vi "logHardpointActuatorInfo.vi"(8 "error in (no error)":errorcluster, 10 "EventHardpointActuatorInfo":T1, 11 "M1M3SAL in":refnum<class "M1M3SAL.lvclass">) -> (0 "error out":errorcluster, 3 "M1M3SAL out":refnum<class "M1M3SAL.lvclass">)   [LabVIEW 2016, in "M1M3SupportCommunicator.lvlib" / "M1M3SAL.lvclass"]
uses:
  M1M3SAL.lvclass
  DataTypes/Topics/EventHardpointActuatorInfo.ctl
  DataTypes/Topics/Parts/Timestamp.ctl
  DataTypes/MessageHeader.ctl
  DataTypes/MessageTypes.ctl
  DataTypes/MessageTopics.ctl
  M1M3SAL.lvclass/M1M3SAL.ctl
  writeU8.vi
  writeSGL.vi
  writeI64.vi
  writeBoolean.vi
  M1M3SupportCommunicator.lvlib
  DataTypes/Topics/M1M3SupportTopics.lvlib
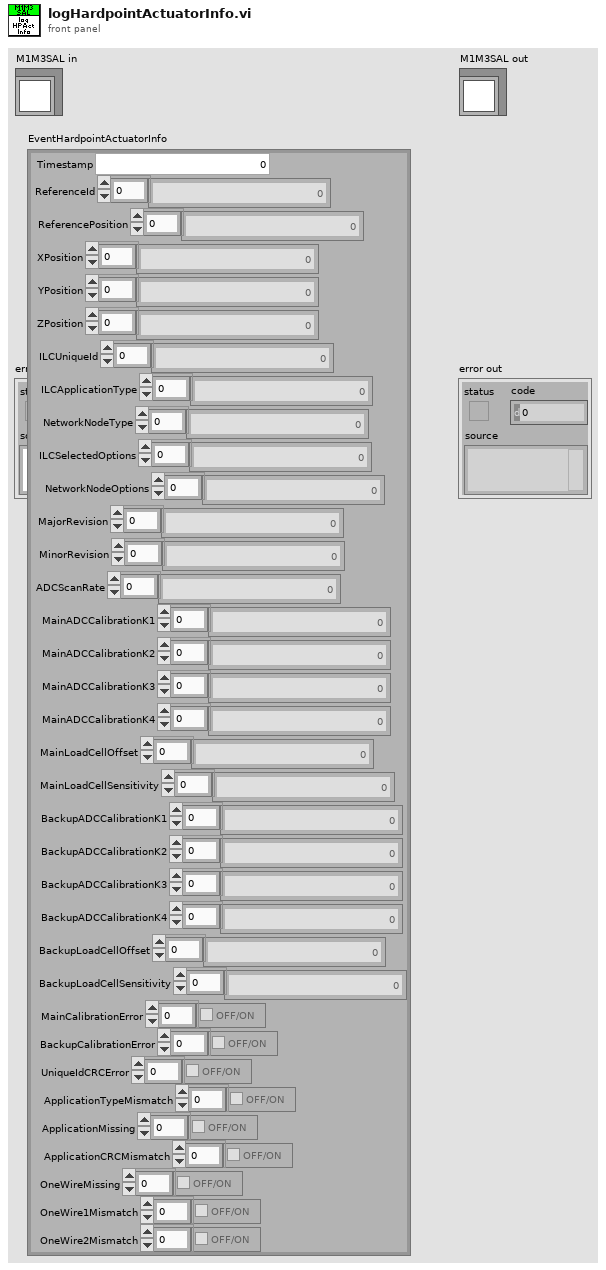
[diagram p1: front panel]
types:
  T1 = typedef "M1M3SupportTopics.lvlib/EventHardpointActuatorInfo.ctl" = cluster{"Timestamp":T2, "ReferenceId":i32[], "ReferencePosition":i32[], "XPosition":sgl[], "YPosition":sgl[], "ZPosition":sgl[], "ILCUniqueId":i64[], "ILCApplicationType":u8[], "NetworkNodeType":u8[], "ILCSelectedOptions":u8[], "NetworkNodeOptions":u8[], "MajorRevision":u8[], "MinorRevision":u8[], "ADCScanRate":u8[], "MainADCCalibrationK1":sgl[], "MainADCCalibrationK2":sgl[], "MainADCCalibrationK3":sgl[], "MainADCCalibrationK4":sgl[], "MainLoadCellOffset":sgl[], "MainLoadCellSensitivity":sgl[], "BackupADCCalibrationK1":sgl[], "BackupADCCalibrationK2":sgl[], "BackupADCCalibrationK3":sgl[], "BackupADCCalibrationK4":sgl[], "BackupLoadCellOffset":sgl[], "BackupLoadCellSensitivity":sgl[], "MainCalibrationError":bool[], "BackupCalibrationError":bool[], "UniqueIdCRCError":bool[], "ApplicationTypeMismatch":bool[], "ApplicationMissing":bool[], "ApplicationCRCMismatch":bool[], "OneWireMissing":bool[], "OneWire1Mismatch":bool[], "OneWire2Mismatch":bool[]}
  T2 = typedef "M1M3SupportTopics.lvlib/Timestamp.ctl" = dbl
  T3 = typedef "M1M3SupportCommunicator.lvlib/MessageHeader.ctl" = cluster{"Type":T4, "Topic":T5, "Size":i32}
  T4 = typedef "M1M3SupportCommunicator.lvlib/MessageTypes.ctl" = enum8{"None", "PutSample", "GetNextSample", "LogEvent", "GetEvent", "IssueCommand", "CommandId", "WaitForCompletion", "AcceptCommand", "AckCommand"}
  T5 = typedef "M1M3SupportCommunicator.lvlib/MessageTopics.ctl" = enum8{"None", "ForceActuatorData", "MirrorForceData", "HardpointData", "AirData", "DynamicData", "FPGAData", "IMSData", "ForceActuatorStatus", "ElevationData", "HardpointStatus", "HardpointActuatorChase", "AirStatus", "ForceActuatorSafetyChecks", "ForceActuatorTest", "ActuatorBroadcastCounter", "StatusChecks", "CellChecks", "HardpointActuatorBreakaway", "RaiseMirrorComplete", "ILCCommunication", "ElevationAngleChecks", "DetailedState", "ServoLoops", "ForceActuatorInfo", "LowerMirrorComplete", "HardpointActuatorInfo", "SettingsApplied", "ErrorCode", "StartupChecks", "SummaryState", "SettingVersions", "ActuatorTestStatus", "AppliedSettingsMatchStart", "Enable", "EnterMaintenance", "Standby", "AbortLowerM1M3", "ApplyAberrationByForces", "ApplyAOSCorrectionByBendingModes", "ClearAOSCorrection", "Start", "RaiseM1M3", "TestForceActuator", "LowerM1M3", "ApplyAOSCorrectionByForces", "Disable", "ApplyAberationByBendingMode", "TestHardpoint", "ManipulateM1M3", "ClearAberration", "Exit", "TestAir", "AbortRaiseM1M3", "MoveHardpointActuators", "ExitMaintenance", "Shutdown"}
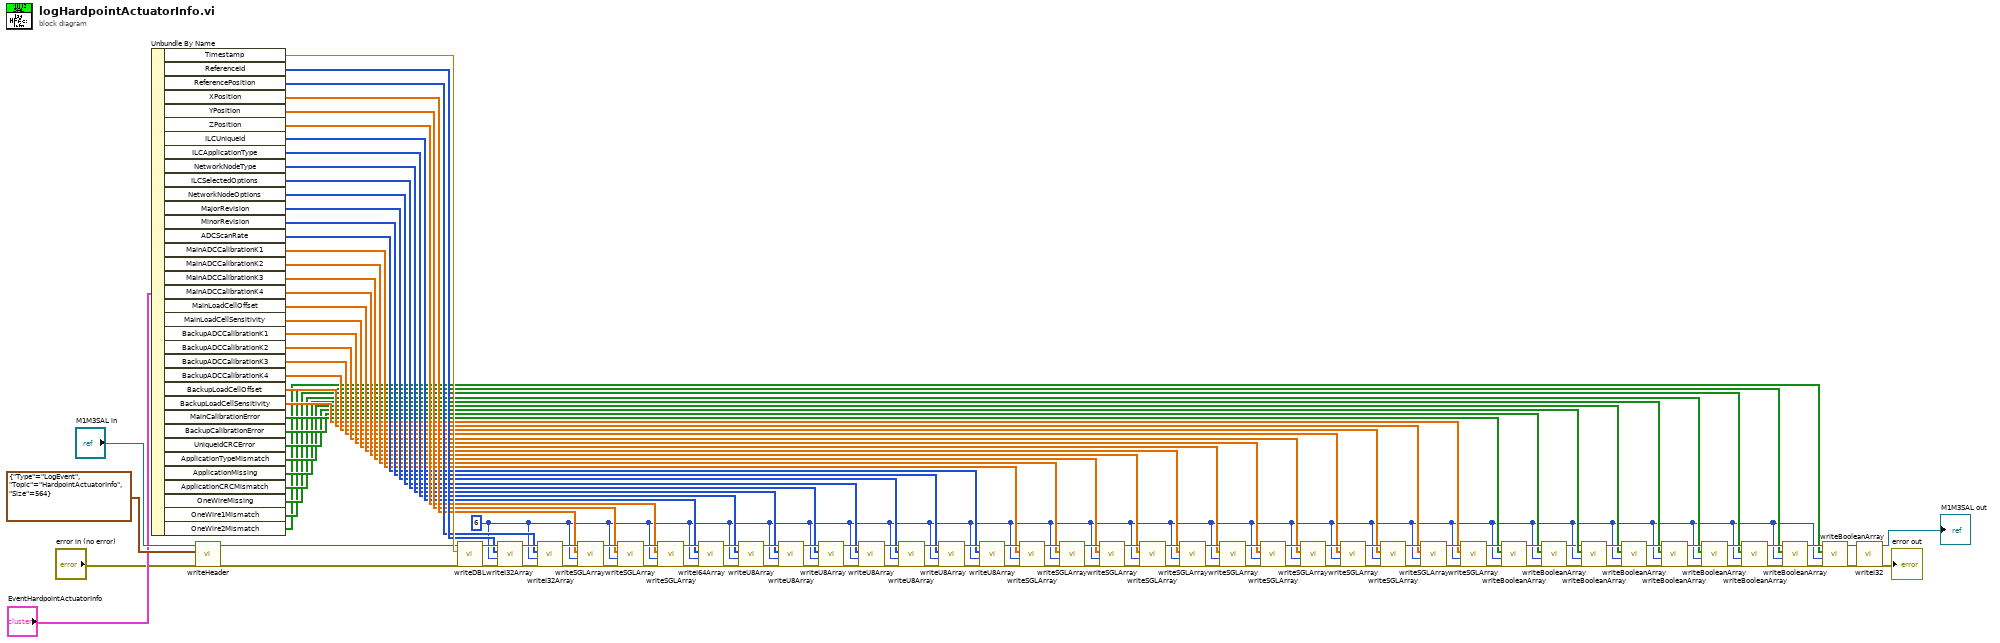
[diagram p0: block diagram]
diagram:
  w4 = 6
  n1 = Unbundle By Name("EventHardpointActuatorInfo") -> ("Timestamp"=w41:T2, "ReferenceId"=w40:i32[], "ReferencePosition"=w39:i32[], "XPosition"=w38:sgl[], "YPosition"=w37:sgl[], "ZPosition"=w36:sgl[], "ILCUniqueId"=w35:i64[], "ILCApplicationType"=w34:u8[], "NetworkNodeType"=w33:u8[], "ILCSelectedOptions"=w32:u8[], "NetworkNodeOptions"=w31:u8[], "MajorRevision"=w30:u8[], "MinorRevision"=w29:u8[], "ADCScanRate"=w28:u8[], "MainADCCalibrationK1"=w27:sgl[], "MainADCCalibrationK2"=w26:sgl[], "MainADCCalibrationK3"=w25:sgl[], "MainADCCalibrationK4"=w24:sgl[], "MainLoadCellOffset"=w23:sgl[], "MainLoadCellSensitivity"=w22:sgl[], "BackupADCCalibrationK1"=w21:sgl[], "BackupADCCalibrationK2"=w20:sgl[], "BackupADCCalibrationK3"=w19:sgl[], "BackupADCCalibrationK4"=w18:sgl[], "BackupLoadCellOffset"=w17:sgl[], "BackupLoadCellSensitivity"=w16:sgl[], "MainCalibrationError"=w15:bool[], "BackupCalibrationError"=w14:bool[], "UniqueIdCRCError"=w13:bool[], "ApplicationTypeMismatch"=w10:bool[], "ApplicationMissing"=w9:bool[], "ApplicationCRCMismatch"=w8:bool[], "OneWireMissing"=w7:bool[], "OneWire1Mismatch"=w6:bool[], "OneWire2Mismatch"=w5:bool[])
  n2 = call "writeHeader.vi"("error in (no error)"="error in (no error)", "MessageHeader"=T3 {"Type"=enum."LogEvent", "Topic"=enum."HardpointActuatorInfo", "Size"=564}, "M1M3SAL in"="M1M3SAL in") -> ("error out"=w2:errorcluster, "M1M3SAL out"=w3:refnum<class "M1M3SAL.lvclass">)  [unwired: 7 in]
  n3 = call "writeDBL.vi"("error in (no error)"=w2, "Input"=w41, "M1M3SAL in"=w3) -> ("error out"=w107:errorcluster, "M1M3SAL out"=w106:refnum<class "M1M3SAL.lvclass">)  [unwired: 7 in]
  n4 = call "writeI32Array.vi"("error in (no error)"=w107, "Length"=w4, "Input"=w40, "M1M3SAL in"=w106) -> ("error out"=w111:errorcluster, "M1M3SAL out"=w110:refnum<class "M1M3SAL.lvclass">)  [unwired: 6 in]
  n5 = call "writeI32Array.vi"("error in (no error)"=w111, "Length"=w4, "Input"=w39, "M1M3SAL in"=w110) -> ("error out"=w108:errorcluster, "M1M3SAL out"=w109:refnum<class "M1M3SAL.lvclass">)  [unwired: 6 in]
  n6 = call "writeSGLArray.vi"("error in (no error)"=w108, "Length"=w4, "Input"=w38, "M1M3SAL in"=w109) -> ("error out"=w105:errorcluster, "M1M3SAL out"=w104:refnum<class "M1M3SAL.lvclass">)  [unwired: 6 in]
  n7 = call "writeSGLArray.vi"("error in (no error)"=w105, "Length"=w4, "Input"=w37, "M1M3SAL in"=w104) -> ("error out"=w103:errorcluster, "M1M3SAL out"=w102:refnum<class "M1M3SAL.lvclass">)  [unwired: 6 in]
  n8 = call "writeSGLArray.vi"("error in (no error)"=w103, "Length"=w4, "Input"=w36, "M1M3SAL in"=w102) -> ("error out"=w100:errorcluster, "M1M3SAL out"=w101:refnum<class "M1M3SAL.lvclass">)  [unwired: 6 in]
  n9 = call "writeI64Array.vi"("error in (no error)"=w100, "Length"=w4, "Input"=w35, "M1M3SAL in"=w101) -> ("error out"=w98:errorcluster, "M1M3SAL out"=w99:refnum<class "M1M3SAL.lvclass">)  [unwired: 6 in]
  n10 = call "writeU8Array.vi"("error in (no error)"=w98, "Length"=w4, "Input"=w34, "M1M3SAL in"=w99) -> ("error out"=w97:errorcluster, "M1M3SAL out"=w96:refnum<class "M1M3SAL.lvclass">)  [unwired: 6 in]
  n11 = call "writeU8Array.vi"("error in (no error)"=w97, "Length"=w4, "Input"=w33, "M1M3SAL in"=w96) -> ("error out"=w95:errorcluster, "M1M3SAL out"=w94:refnum<class "M1M3SAL.lvclass">)  [unwired: 6 in]
  n12 = call "writeU8Array.vi"("error in (no error)"=w95, "Length"=w4, "Input"=w32, "M1M3SAL in"=w94) -> ("error out"=w93:errorcluster, "M1M3SAL out"=w92:refnum<class "M1M3SAL.lvclass">)  [unwired: 6 in]
  n13 = call "writeU8Array.vi"("error in (no error)"=w93, "Length"=w4, "Input"=w31, "M1M3SAL in"=w92) -> ("error out"=w91:errorcluster, "M1M3SAL out"=w90:refnum<class "M1M3SAL.lvclass">)  [unwired: 6 in]
  n14 = call "writeU8Array.vi"("error in (no error)"=w91, "Length"=w4, "Input"=w30, "M1M3SAL in"=w90) -> ("error out"=w89:errorcluster, "M1M3SAL out"=w88:refnum<class "M1M3SAL.lvclass">)  [unwired: 6 in]
  n15 = call "writeU8Array.vi"("error in (no error)"=w89, "Length"=w4, "Input"=w29, "M1M3SAL in"=w88) -> ("error out"=w87:errorcluster, "M1M3SAL out"=w86:refnum<class "M1M3SAL.lvclass">)  [unwired: 6 in]
  n16 = call "writeU8Array.vi"("error in (no error)"=w87, "Length"=w4, "Input"=w28, "M1M3SAL in"=w86) -> ("error out"=w85:errorcluster, "M1M3SAL out"=w84:refnum<class "M1M3SAL.lvclass">)  [unwired: 6 in]
  n17 = call "writeSGLArray.vi"("error in (no error)"=w85, "Length"=w4, "Input"=w27, "M1M3SAL in"=w84) -> ("error out"=w83:errorcluster, "M1M3SAL out"=w82:refnum<class "M1M3SAL.lvclass">)  [unwired: 6 in]
  n18 = call "writeSGLArray.vi"("error in (no error)"=w83, "Length"=w4, "Input"=w26, "M1M3SAL in"=w82) -> ("error out"=w81:errorcluster, "M1M3SAL out"=w80:refnum<class "M1M3SAL.lvclass">)  [unwired: 6 in]
  n19 = call "writeSGLArray.vi"("error in (no error)"=w81, "Length"=w4, "Input"=w25, "M1M3SAL in"=w80) -> ("error out"=w79:errorcluster, "M1M3SAL out"=w78:refnum<class "M1M3SAL.lvclass">)  [unwired: 6 in]
  n20 = call "writeSGLArray.vi"("error in (no error)"=w79, "Length"=w4, "Input"=w24, "M1M3SAL in"=w78) -> ("error out"=w77:errorcluster, "M1M3SAL out"=w76:refnum<class "M1M3SAL.lvclass">)  [unwired: 6 in]
  n21 = call "writeSGLArray.vi"("error in (no error)"=w77, "Length"=w4, "Input"=w23, "M1M3SAL in"=w76) -> ("error out"=w75:errorcluster, "M1M3SAL out"=w74:refnum<class "M1M3SAL.lvclass">)  [unwired: 6 in]
  n22 = call "writeSGLArray.vi"("error in (no error)"=w75, "Length"=w4, "Input"=w22, "M1M3SAL in"=w74) -> ("error out"=w73:errorcluster, "M1M3SAL out"=w72:refnum<class "M1M3SAL.lvclass">)  [unwired: 6 in]
  n23 = call "writeSGLArray.vi"("error in (no error)"=w73, "Length"=w4, "Input"=w21, "M1M3SAL in"=w72) -> ("error out"=w71:errorcluster, "M1M3SAL out"=w70:refnum<class "M1M3SAL.lvclass">)  [unwired: 6 in]
  n24 = call "writeSGLArray.vi"("error in (no error)"=w71, "Length"=w4, "Input"=w20, "M1M3SAL in"=w70) -> ("error out"=w69:errorcluster, "M1M3SAL out"=w68:refnum<class "M1M3SAL.lvclass">)  [unwired: 6 in]
  n25 = call "writeSGLArray.vi"("error in (no error)"=w69, "Length"=w4, "Input"=w19, "M1M3SAL in"=w68) -> ("error out"=w67:errorcluster, "M1M3SAL out"=w66:refnum<class "M1M3SAL.lvclass">)  [unwired: 6 in]
  n26 = call "writeSGLArray.vi"("error in (no error)"=w67, "Length"=w4, "Input"=w18, "M1M3SAL in"=w66) -> ("error out"=w65:errorcluster, "M1M3SAL out"=w64:refnum<class "M1M3SAL.lvclass">)  [unwired: 6 in]
  n27 = call "writeSGLArray.vi"("error in (no error)"=w65, "Length"=w4, "Input"=w17, "M1M3SAL in"=w64) -> ("error out"=w63:errorcluster, "M1M3SAL out"=w62:refnum<class "M1M3SAL.lvclass">)  [unwired: 6 in]
  n28 = call "writeSGLArray.vi"("error in (no error)"=w63, "Length"=w4, "Input"=w16, "M1M3SAL in"=w62) -> ("error out"=w60:errorcluster, "M1M3SAL out"=w61:refnum<class "M1M3SAL.lvclass">)  [unwired: 6 in]
  n29 = call "writeBooleanArray.vi"("error in (no error)"=w60, "Length"=w4, "Input"=w15, "M1M3SAL in"=w61) -> ("error out"=w59:errorcluster, "M1M3SAL out"=w58:refnum<class "M1M3SAL.lvclass">)  [unwired: 6 in]
  n30 = call "writeBooleanArray.vi"("error in (no error)"=w59, "Length"=w4, "Input"=w14, "M1M3SAL in"=w58) -> ("error out"=w11:errorcluster, "M1M3SAL out"=w12:refnum<class "M1M3SAL.lvclass">)  [unwired: 6 in]
  n31 = call "writeBooleanArray.vi"("error in (no error)"=w11, "Length"=w4, "Input"=w13, "M1M3SAL in"=w12) -> ("error out"=w57:errorcluster, "M1M3SAL out"=w56:refnum<class "M1M3SAL.lvclass">)  [unwired: 6 in]
  n32 = call "writeBooleanArray.vi"("error in (no error)"=w57, "Length"=w4, "Input"=w10, "M1M3SAL in"=w56) -> ("error out"=w55:errorcluster, "M1M3SAL out"=w54:refnum<class "M1M3SAL.lvclass">)  [unwired: 6 in]
  n33 = call "writeBooleanArray.vi"("error in (no error)"=w55, "Length"=w4, "Input"=w9, "M1M3SAL in"=w54) -> ("error out"=w50:errorcluster, "M1M3SAL out"=w51:refnum<class "M1M3SAL.lvclass">)  [unwired: 6 in]
  n34 = call "writeBooleanArray.vi"("error in (no error)"=w50, "Length"=w4, "Input"=w8, "M1M3SAL in"=w51) -> ("error out"=w53:errorcluster, "M1M3SAL out"=w52:refnum<class "M1M3SAL.lvclass">)  [unwired: 6 in]
  n35 = call "writeBooleanArray.vi"("error in (no error)"=w53, "Length"=w4, "Input"=w7, "M1M3SAL in"=w52) -> ("error out"=w49:errorcluster, "M1M3SAL out"=w48:refnum<class "M1M3SAL.lvclass">)  [unwired: 6 in]
  n36 = call "writeBooleanArray.vi"("error in (no error)"=w49, "Length"=w4, "Input"=w6, "M1M3SAL in"=w48) -> ("error out"=w47:errorcluster, "M1M3SAL out"=w46:refnum<class "M1M3SAL.lvclass">)  [unwired: 6 in]
  n37 = call "writeBooleanArray.vi"("error in (no error)"=w47, "Length"=w4, "Input"=w5, "M1M3SAL in"=w46) -> ("error out"=w44:errorcluster, "M1M3SAL out"=w45:refnum<class "M1M3SAL.lvclass">)  [unwired: 6 in]
  n38 = call "writeI32.vi"("error in (no error)"=w44, "M1M3SAL in"=w45) -> ("error out"=→"error out":errorcluster, "M1M3SAL out"=→"M1M3SAL out":refnum<class "M1M3SAL.lvclass">)  [unwired: 8 in]
